vi "Read_Sku.vi"(8 "SKU":string) -> (0 "Recipe":string)   [LabVIEW 2017]
panel:
  out "元素索引":i32
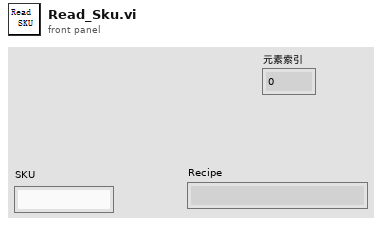
[diagram p1: front panel]
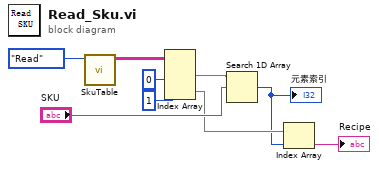
[diagram p0: block diagram]
diagram:
  n1 = call "SkuTable.vi"("Step"=enum16{"Initial", "Write", "Read"}."Read") -> ("Tabledata Out"=w8:string[][])  [unwired: 9 in, 1 out]
  n2 = Index Array(array=w8, index (col) #1=0 ("禁用的索引 (列)"), index (col) #2=1 ("索引 (列)")) -> (element #1=w6:string[], element #2=w3:string[])  [unwired: 2 in]
  n3 = Search 1D Array(1D array=w6, element="SKU") -> (index of element=w2:i32)  [unwired: 1 in]
  "元素索引" <- w2
  n4 = Index Array(array=w3, index=w2) -> (element=→"Recipe":string)
